vi "CreateDirectory.vi"(5 "Relative Path":path=path "config/images", 6 "error in":errorcluster, 9 "PythonConverter_GUI in":refnum<class "PythonConverter_GUI.lvclass">) -> (0 "error out":errorcluster, 3 "PythonConverter_GUI out":refnum<class "PythonConverter_GUI.lvclass">, 4 "Path":path)   [LabVIEW 2014, in "Raspberry Pi Compatible Compiler for LabVIEW.lvlib" / "PythonConverter_GUI.lvclass"]
uses:
  PythonConverter_GUI.lvclass
  PythonConverter_GUI.lvclass/PythonConverter_GUI.ctl
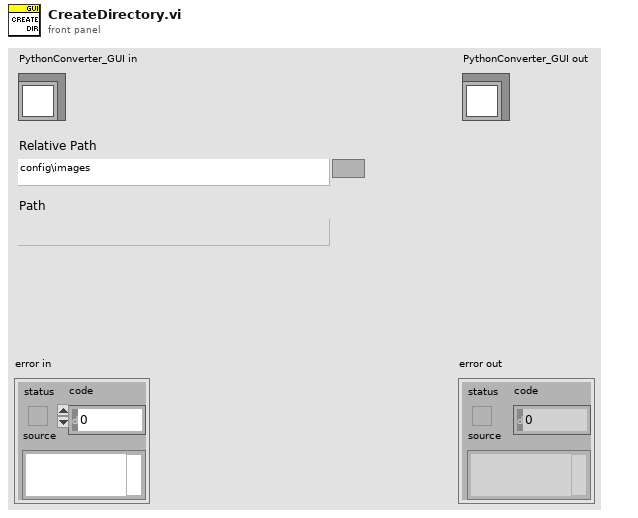
[diagram p1: front panel]
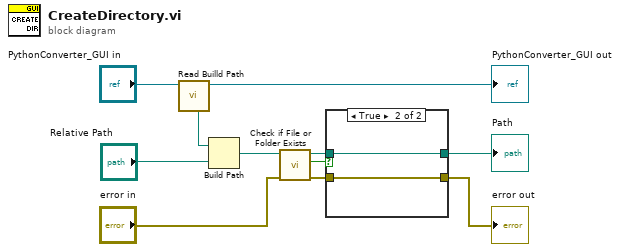
[diagram p0: block diagram]
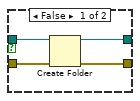
[diagram p2: hidden frame]
diagram:
  n1 = call "Read Builld Path.vi"("PythonConverter_GUI in"="PythonConverter_GUI in") -> ("PythonConverter_GUI out"=→"PythonConverter_GUI out":refnum<class "PythonConverter_GUI.lvclass">, "Builld Path"=w10:path)  [unwired: 7 in]
  n2 = Build Path(base path=w10, name or relative path="Relative Path") -> (appended path=w8:path)
  n3 = call <vilib>:"Check if File or Folder Exists.vi"("error in (no error)"="error in", "path"=w8) -> ("error out"=w6:errorcluster, "file or folder exists?"=w5:bool, "dup path"=w7:path)  [unwired: 7 in]
  n4 = case shown="True" w5 {
    tunnel: w7 -> [w15 w16]
    tunnel: w6 -> [w14 w17]
    tunnel: [w13 w17] -> w3
    tunnel: [w12 w16] -> w2
    frame False {
      n5 = Create Folder(path (use dialog)=w15, error in=w14) -> (created path=w12:path, error out=w13:errorcluster)  [unwired: 1 in, 1 out]
    }
    frame True {
    }
  }
  "error out" <- w3
  "Path" <- w2
